vi "openAnalysisViewer.vi"(8 "error in (no error)":errorcluster, 10 "whichViewer":string, 11 "ImageStreamViewer in":refnum<class "ImageStreamViewer.lvclass">) -> (0 "error out":errorcluster, 3 "ImageStreamViewer out":refnum<class "ImageStreamViewer.lvclass">)   [LabVIEW 2011, in "Views.lvlib" / "Camera.lvlib" / "ImageStreamViewer.lvclass"]
uses:
  ImageStreamViewer.lvclass
  AnalysisResultsViewer/AnalysisResultsViewer.lvclass
  ImageStreamViewer.lvclass/ImageStreamViewer.ctl
  Tools/Filing/FileSystem/FileSystem.lvclass
  AnalysisResultsViewer/FringeTestingViewer/FringeTestingViewer.lvclass
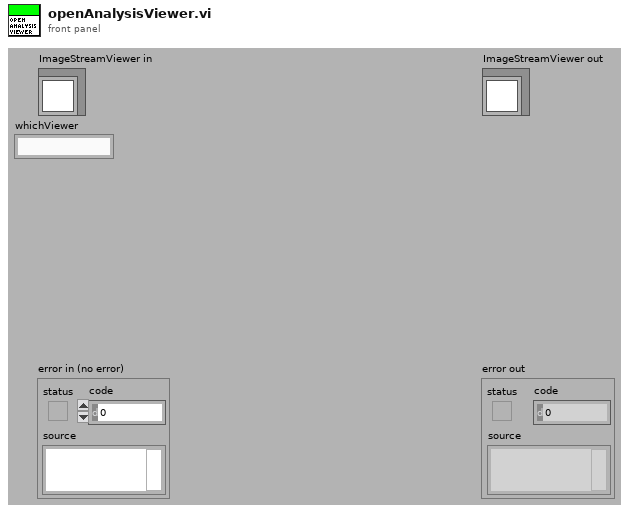
[diagram p1: front panel]
types:
  T1 = enum32{"Invalid", "Standard", "Closed", "Hidden", "Minimized", "Maximized"}
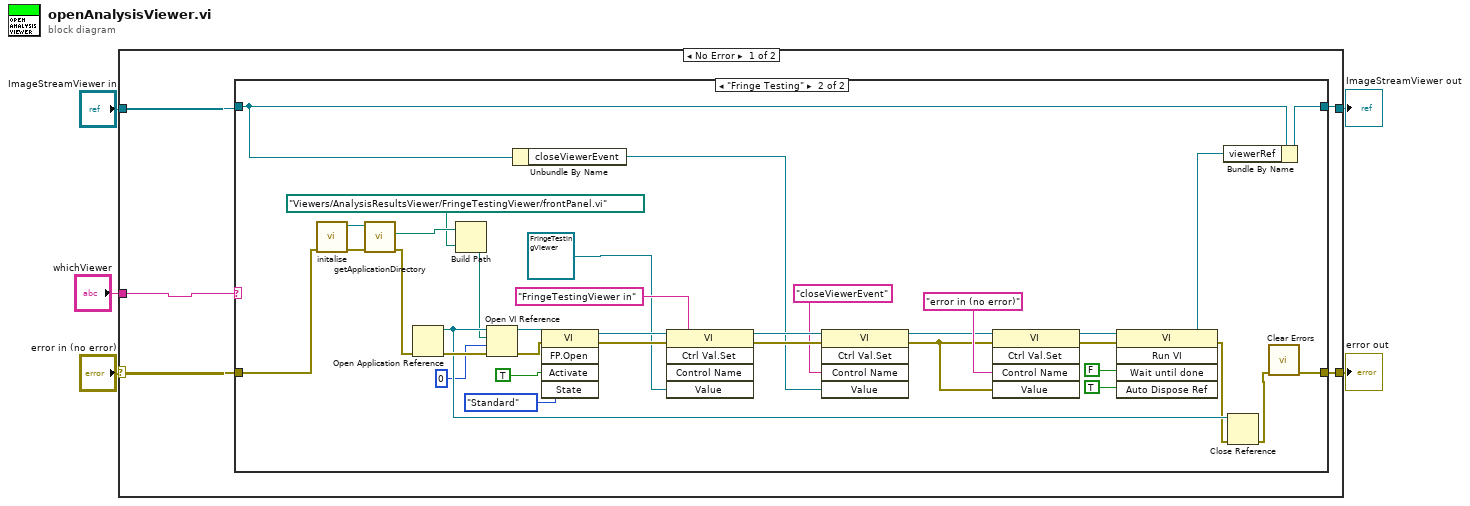
[diagram p0: block diagram]
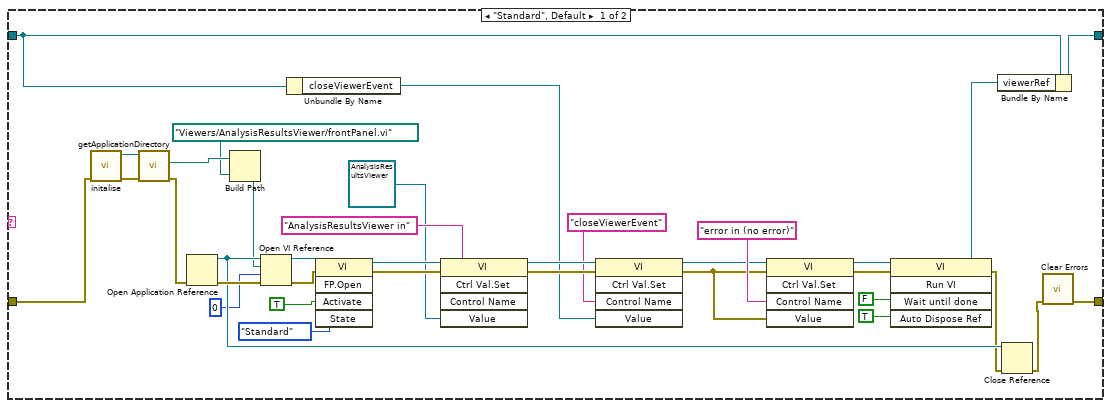
[diagram p2: hidden frame]
diagram:
  n1 = case shown="No Error" "error in (no error)" {
    selector: "error in (no error)" -> [w10 w82]
    tunnel: [w9 w82] -> w4
    tunnel: [w7 w81] -> w2
    tunnel: "ImageStreamViewer in" -> [w8 w81]
    tunnel: "whichViewer" -> [w6 _]
    frame No Error {
      n2 = case shown="\"Fringe Testing\"" w6 {
        tunnel: w10 -> [w23 w58]
        tunnel: [w21 w56] -> w9
        tunnel: w8 -> [w20 w55]
        tunnel: [w18 w53] -> w7
        frame "Standard", Default {
          n3 = call "initalise.vi"("error in (no error)"=w23) -> ("error out"=w28:errorcluster, "FileSystem out"=w27:refnum<class "FileSystem.lvclass">)  [unwired: 9 in]
          n4 = call-dynamic "getApplicationDirectory.vi"("error in (no error)"=w28, "FileSystem.lvclass in"=w27) -> ("error out"=w26:errorcluster, "ApplicationDirectory"=w30:path)  [unwired: 7 in, 1 out]
          n5 = Open Application Reference(8:w26) -> (0:w42:errorcluster, 3:w41:refnum<vi>)  [unwired: 3 in]
          n6 = Build Path(base path=w30, name or relative path=path "Viewers/AnalysisResultsViewer/frontPanel.vi" ("vi path")) -> (appended path=w25:path)
          n7 = Open VI Reference(application reference (local)=w41, vi path=w25, options=0, error in (no error)=w42) -> (vi reference=w37:refnum<vi>, error out=w36:errorcluster)  [unwired: 2 in]
          n8 = Unbundle By Name(w20) -> ("closeViewerEvent"=w14:refnum<user-event>)
          n9 = invoke class="VI" method="FP.Open"(reference=w37, error in=w36, "Activate"=TRUE, "State"=T1."Standard") -> (reference out=w35:refnum<vi>, error out=w34:errorcluster)  [unwired: 1 in, 3 out]
          n10 = invoke class="VI" method="Ctrl Val.Set"(reference=w35, error in=w34, "Control Name"="AnalysisResultsViewer in", "Value"=refnum<class "AnalysisResultsViewer.lvclass"> refnum ("AnalysisResultsViewer in")) -> (reference out=w17:refnum<vi>, error out=w16:errorcluster)  [unwired: 1 in, 3 out]
          n11 = invoke class="VI" method="Ctrl Val.Set"(reference=w17, error in=w16, "Control Name"="closeViewerEvent", "Value"=w14) -> (reference out=w15:refnum<vi>, error out=w12:errorcluster)  [unwired: 1 in, 3 out]
          n12 = invoke class="VI" method="Ctrl Val.Set"(reference=w15, error in=w12, "Control Name"="error in (no error)", "Value"=w12) -> (reference out=w39:refnum<vi>, error out=w38:errorcluster)  [unwired: 1 in, 3 out]
          n13 = invoke class="VI" method="Run VI"(reference=w39, error in=w38, "Wait until done"=FALSE, "Auto Dispose Ref"=TRUE) -> (reference out=w19:refnum<vi>, error out=w40:errorcluster)  [unwired: 1 in, 3 out]
          n14 = Bundle By Name(cluster=w20, "viewerRef"=w19) -> (w18:refnum<class "ImageStreamViewer.lvclass">)
          n15 = Close Reference(reference=w41, error in (no error)=w40) -> (error out=w22:errorcluster)
          n16 = call <vilib>:"Clear Errors.vi"("error in (no error)"=w22) -> ("error out"=w21:errorcluster)  [unwired: 6 in]
        }
        frame "Fringe Testing" {
          n17 = call "initalise.vi"("error in (no error)"=w58) -> ("error out"=w63:errorcluster, "FileSystem out"=w62:refnum<class "FileSystem.lvclass">)  [unwired: 9 in]
          n18 = call-dynamic "getApplicationDirectory.vi"("error in (no error)"=w63, "FileSystem.lvclass in"=w62) -> ("error out"=w61:errorcluster, "ApplicationDirectory"=w65:path)  [unwired: 7 in, 1 out]
          n19 = Open Application Reference(8:w61) -> (0:w77:errorcluster, 3:w76:refnum<vi>)  [unwired: 3 in]
          n20 = Build Path(base path=w65, name or relative path=path "Viewers/AnalysisResultsViewer/FringeTestingViewer/frontPanel.vi" ("vi path")) -> (appended path=w60:path)
          n21 = Open VI Reference(application reference (local)=w76, vi path=w60, options=0, error in (no error)=w77) -> (vi reference=w72:refnum<vi>, error out=w71:errorcluster)  [unwired: 2 in]
          n22 = Unbundle By Name(w55) -> ("closeViewerEvent"=w49:refnum<user-event>)
          n23 = invoke class="VI" method="FP.Open"(reference=w72, error in=w71, "Activate"=TRUE, "State"=T1."Standard") -> (reference out=w70:refnum<vi>, error out=w69:errorcluster)  [unwired: 1 in, 3 out]
          n24 = invoke class="VI" method="Ctrl Val.Set"(reference=w70, error in=w69, "Control Name"="FringeTestingViewer in", "Value"=refnum<class "FringeTestingViewer.lvclass"> refnum ("Views.lvlib:Camera.lvlib:FringeTestingViewer.lvclass")) -> (reference out=w52:refnum<vi>, error out=w51:errorcluster)  [unwired: 1 in, 3 out]
          n25 = invoke class="VI" method="Ctrl Val.Set"(reference=w52, error in=w51, "Control Name"="closeViewerEvent", "Value"=w49) -> (reference out=w50:refnum<vi>, error out=w47:errorcluster)  [unwired: 1 in, 3 out]
          n26 = invoke class="VI" method="Ctrl Val.Set"(reference=w50, error in=w47, "Control Name"="error in (no error)", "Value"=w47) -> (reference out=w74:refnum<vi>, error out=w73:errorcluster)  [unwired: 1 in, 3 out]
          n27 = invoke class="VI" method="Run VI"(reference=w74, error in=w73, "Wait until done"=FALSE, "Auto Dispose Ref"=TRUE) -> (reference out=w54:refnum<vi>, error out=w75:errorcluster)  [unwired: 1 in, 3 out]
          n28 = Bundle By Name(cluster=w55, "viewerRef"=w54) -> (w53:refnum<class "ImageStreamViewer.lvclass">)
          n29 = Close Reference(reference=w76, error in (no error)=w75) -> (error out=w57:errorcluster)
          n30 = call <vilib>:"Clear Errors.vi"("error in (no error)"=w57) -> ("error out"=w56:errorcluster)  [unwired: 6 in]
        }
      }
    }
    frame Error {
    }
  }
  "error out" <- w4
  "ImageStreamViewer out" <- w2
